vi "split_string.vi"(8 "error in (no error)":errorcluster, 10 "delimiter":string, 11 "input string":string) -> (0 "error out":errorcluster, 3 "substrings":string[](array[string]))   [LabVIEW 2010]
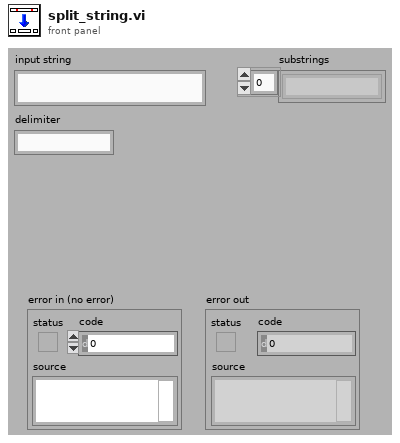
[diagram p1: front panel]
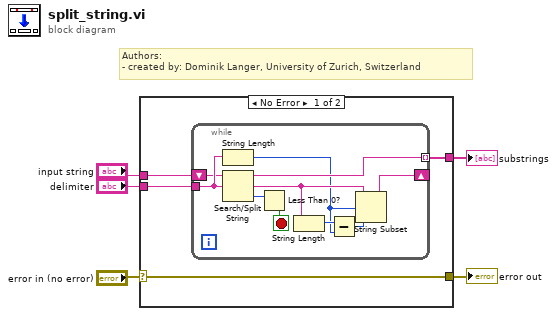
[diagram p0: block diagram]
diagram:
  # "Authors: \n- created by: Dominik Langer, University of Zurich, Switzerland"
  n1 = case shown="No Error" "error in (no error)" {
    selector: "error in (no error)" -> [w8 w20]
    tunnel: "delimiter" -> [w9 _]
    tunnel: [w8 w20] -> w3
    tunnel: "input string" -> [w7 _]
    tunnel: [w6 _] -> w1
    frame No Error {
      n2 = while {
        tunnel: w9 -> [w17]
        tunnel: [w15] -> w6 mode=indexing
        shift-right: [w13] -> _
        shift-left: w7 -> [w16]
        stop <- w10 stop-if-true
        n3 = String Length(string=w17) -> (length=w11:i32)
        n4 = Search/Split String(string=w16, search string/char (-)=w17) -> (substring before match=w15:string, match + rest of string=w19:string, offset of match=w14:i32)  [unwired: 1 in]
        n5 = Less Than 0?(x=w14) -> (x < 0?=w10:bool)
        n6 = String Length(string=w19) -> (length=w12:i32)
        n7 = Subtract(x=w12, y=w11) -> (x-y=w18:i32)
        n8 = String Subset(string=w19, offset (0)=w11, length (rest)=w18) -> (substring=w13:string)
      }
    }
    frame Error {
    }
  }
  "error out" <- w3
  "substrings" <- w1
